vi "_CSMObj-Obtain.vi"(7 "Allowed Messages(Empty for all)":string[](array[string]), 8 "Error in":errorcluster caption="Error in (no error)", 11 "Requested Name":string) -> (0 "Error out":errorcluster, 3 "CSMQ out":T1={"Requested Name"="", "Module Name"="", "Mode"=enum."Stand Alone", "Queue"=refnum, "CSM-Data"=refnum, "User Event"=refnum, "Status Change Event"=refnum, "Allowed Messages"=[], "Mode-Data"=refnum, "Group Name"="", "Exit Event"=refnum})   [LabVIEW 2020, in "Communicable State Machine.lvlib"]
uses:
  Communicable State Machine.lvlib
  _CSMObj.ctl
  Priority Queue.lvclass
  _CSM_MODE.ctl
  _CSMObj-Data.ctl
  _CSM Status Change Event Data.ctl
  _CSMObj-ModeData.ctl
  Priority Queue.lvclass/Priority Queue.ctl
  Obtain Priority Queue.vi
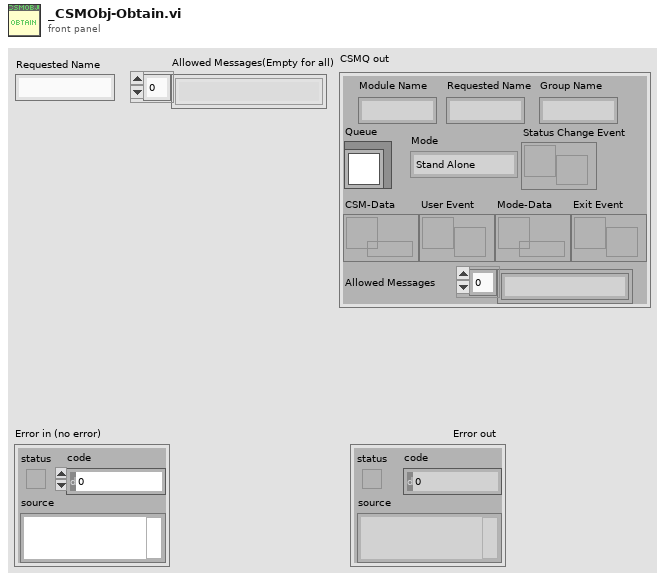
[diagram p1: front panel]
types:
  T1 = typedef "Communicable State Machine.lvlib/_CSMObj.ctl" = cluster{"Requested Name":string, "Module Name":string, "Mode":T2, "Queue":refnum<class "Priority Queue.lvclass">, "CSM-Data":refnum<data-value>, "User Event":refnum<user-event>, "Status Change Event":refnum<user-event>, "Allowed Messages":string[], "Mode-Data":refnum<data-value>, "Group Name":string, "Exit Event":refnum<user-event>}
  T2 = typedef "Communicable State Machine.lvlib/_CSM_MODE.ctl" = enum16{"Not Exist", "Stand Alone", "CSM", "Worker Agent", "Worker", "Chain", "Chain Node"}
  T3 = typedef "Communicable State Machine.lvlib/_CSMObj-ModeData.ctl" = cluster{"Share Count":i32, "Messages of Chain Nodes":cluster{"Module Name":string, "Allowed Messages":string[]}[], "Chain Message Mapping Map":variant}
  T4 = typedef "Communicable State Machine.lvlib/_CSMObj-Data.ctl" = cluster{"RemoteMessge?":bool, "error":errorcluster}
  T5 = typedef "Communicable State Machine.lvlib/_CSM_NAME_REQUEST.ctl" = enum16{"Stand Alone CSM Request", "Normal CSM Request", "Agent Request", "Action Worker Request", "Chain Request", "Chain Node Request"}
  T6 = typedef "Communicable State Machine.lvlib/_CSM Status Change Event Data.ctl" = cluster{"ModuleName":string, "Status":string, "Arguments":string}
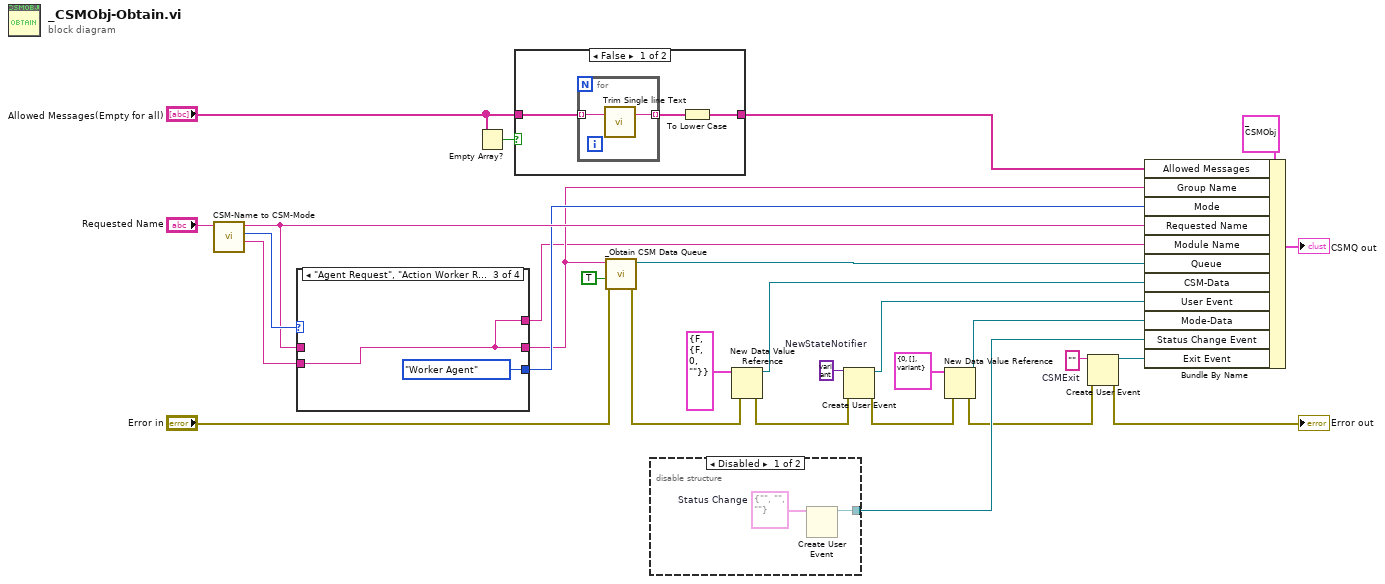
[diagram p0: block diagram]
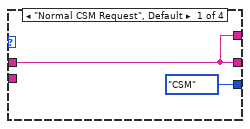
[diagram p2: hidden frame]
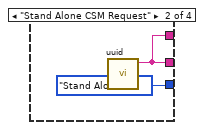
[diagram p3: hidden frame]
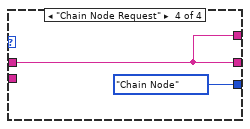
[diagram p4: hidden frame]
diagram:
  w4 = ""  # CSMExit
  w26 = variant  # NewStateNotifier
  n1 = call "CSM-Name to CSM-Mode.vi"("String"="Requested Name") -> ("ParentCSM Name"=w15:string, "CSM Mode"=w13:T5, "Requested Name"=w12:string)  [unwired: 8 in]
  n2 = case shown="\"Agent Request\", \"Action Worker Request\"" w13 {
    tunnel: [w30 w32 w34 w36] -> w7
    tunnel: w12 -> [w30 _ _ w36]
    tunnel: w15 -> [_ _ w34 _]
    tunnel: [_CSM_MODE."CSM" ("Mode") _CSM_MODE."Stand Alone" ("Mode") _CSM_MODE."Worker Agent" ("Mode") _CSM_MODE."Chain Node" ("Mode")] -> w11
    tunnel: [w30 w32 w34 w36] -> w6
    frame "Normal CSM Request", Default {
    }
    frame "Stand Alone CSM Request" {
      n3 = call "uuid.vi"() -> ("UUID"=w32:string)  [unwired: 11 in]
    }
    frame "Agent Request", "Action Worker Request" {
    }
    frame "Chain Node Request" {
    }
  }
  n4 = Empty Array?(array="Allowed Messages(Empty for all)") -> (empty?=w16:bool)
  n5 = case shown="False" w16 {
    tunnel: [w38 w43] -> w18
    tunnel: "Allowed Messages(Empty for all)" -> [w39 w43]
    frame False {
      n6 = for {
        tunnel: [w41] -> w40 mode=indexing
        tunnel: w39 -> [w42] mode=indexing
        n7 = call "Trim Single line Text.vi"("single-line text"=w42) -> ("trimed text"=w41:string)  [unwired: 2 in]
      }
      n8 = To Lower Case(string=w40) -> (all lower case string=w38:string[])
    }
    frame True {
    }
  }
  n9 = call "_Obtain CSM Data Queue.vi"("error in (no error)"="Error in", "create if not found? (T)"=TRUE, "Name"=w7) -> ("error out"=w27:errorcluster, "Priority Queue"=w29:refnum<class "Priority Queue.lvclass">)  [unwired: 6 in, 1 out]
  n10 = disable-structure shown="Disabled" {
    disable-tunnel: [w44 _] -> w23
    frame Disabled {
      w45 = T6 {"ModuleName"="", "Status"="", "Arguments"=""}  # Status Change
      n11 = Create User Event(user event datatype=w45) -> (user event=w44:refnum<user-event>)  [unwired: 1 in, 1 out]
    }
    frame Enabled {
    }
  }
  n12 = New Data Value Reference(data value=T4 {"RemoteMessge?"=FALSE, "error"={"status"=FALSE, "code"=0, "source"=""}} ("CSMObj-Data"), error in=w27) -> (data value reference=w28:refnum<data-value>, error out=w25:errorcluster)
  n13 = Create User Event(user event datatype=w26, error in=w25) -> (user event=w24:refnum<user-event>, error out=w8:errorcluster)
  n14 = New Data Value Reference(data value=T3 {"Share Count"=0, "Messages of Chain Nodes"=[], "Chain Message Mapping Map"=variant} ("CSMObj-Data"), error in=w8) -> (data value reference=w9:refnum<data-value>, error out=w2:errorcluster)
  n15 = Create User Event(user event datatype=w4, error in=w2) -> (user event=w3:refnum<user-event>, error out=→"Error out":errorcluster)
  n16 = Bundle By Name(cluster=T1 {"Requested Name"="", "Module Name"="", "Mode"=enum."Stand Alone", "Queue"=refnum, "CSM-Data"=refnum, "User Event"=refnum, "Status Change Event"=refnum, "Allowed Messages"=[], "Mode-Data"=refnum, "Group Name"="", "Exit Event"=refnum} ("CSMQ in"), "Allowed Messages"=w18, "Group Name"=w7, "Mode"=w11, "Requested Name"=w12, "Module Name"=w6, "Queue"=w29, "CSM-Data"=w28, "User Event"=w24, "Mode-Data"=w9, "Status Change Event"=w23, "Exit Event"=w3) -> (→"CSMQ out":T1)
